vi "SeCrTs-Combo box string Write.vi"(8 "error in (no error)":errorcluster, 10 "Array 2":string[][](array[string]), 11 "Array":refnum<vi>[](array[refnum])) -> (0 "error out":errorcluster)   [LabVIEW 2022 SP3]
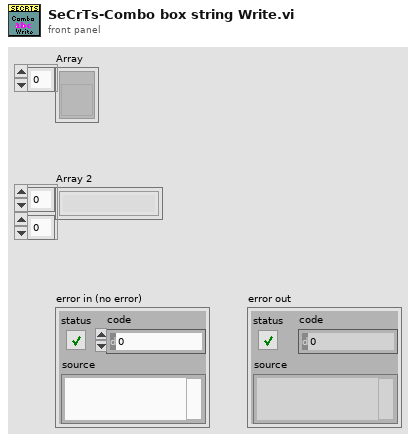
[diagram p1: front panel]
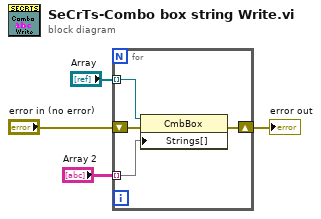
[diagram p0: block diagram]
diagram:
  n1 = for {
    shift-right: [w7] -> w1
    shift-left: "error in (no error)" -> [w8]
    tunnel: "Array 2" -> [w6] mode=indexing
    tunnel: "Array" -> [w5] mode=indexing
    n2 = property on="Property Node" class="CmbBox"(reference=w5, error in=w8, "Strings[]"=w6) -> (error out=w7:errorcluster)  [unwired: 1 out]
  }
  "error out" <- w1
